vi "J1939FullDB.vi"() -> ()   [LabVIEW 2013, in "database file.lvclass"]
uses:
  database file.lvclass
  J1939 Library/Configuration/TypeDefs/J1939 db.ctl
  J1939 Library/Configuration/TypeDefs/J1939 db frame.ctl
  J1939 Library/Configuration/TypeDefs/J1939 db signal.ctl
  J1939 Library/J1939.lvlib
panel:
  in  "default db":T1
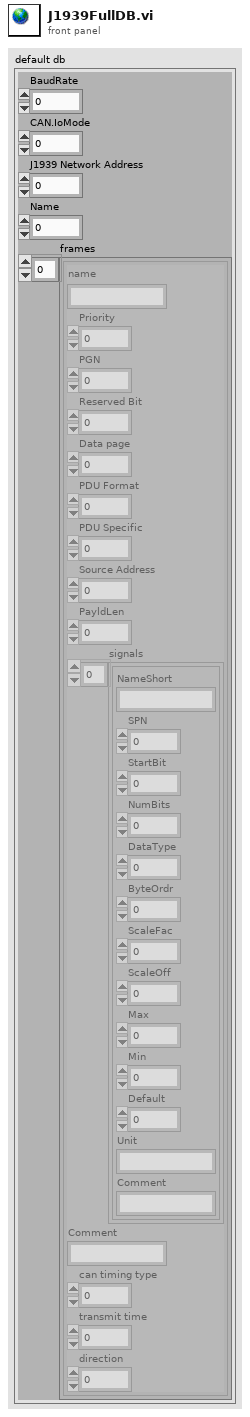
[diagram p1: front panel]
types:
  T1 = typedef "J1939.lvlib/J1939 db.ctl" = cluster{"BaudRate":u32, "CAN.IoMode":u32, "J1939 Network Address":u8, "Name":u64, "frames":T2[]}
  T2 = typedef "J1939.lvlib/J1939 db frame.ctl" = cluster{"name":string, "Priority":u8, "PGN":u32, "Reserved Bit":u8, "Data page":u8, "PDU Format":u8, "PDU Specific":u8, "Source Address":u8, "PayldLen":u32, "signals":T3[], "Comment":string, "can timing type":u32, "transmit time":dbl, "direction":u16}
  T3 = typedef "J1939.lvlib/J1939 db signal.ctl" = cluster{"NameShort":string, "SPN":i32, "StartBit":u32, "NumBits":u32, "DataType":u32, "ByteOrdr":u32, "ScaleFac":dbl, "ScaleOff":dbl, "Max":dbl, "Min":dbl, "Default":dbl, "Unit":string, "Comment":string}
diagram:
